vi "Draw.vi"(8 "error in (no error)":errorcluster, 11 "Link in":refnum<class "Link.lvclass">) -> (0 "error out":errorcluster, 2 "Picture":picture, 3 "Link out":refnum<class "Link.lvclass">)   [LabVIEW 2017, in "LV Image Editor Framework.lvlib" / "Link.lvclass"]
uses:
  Link.lvclass
  Line/Line.lvclass
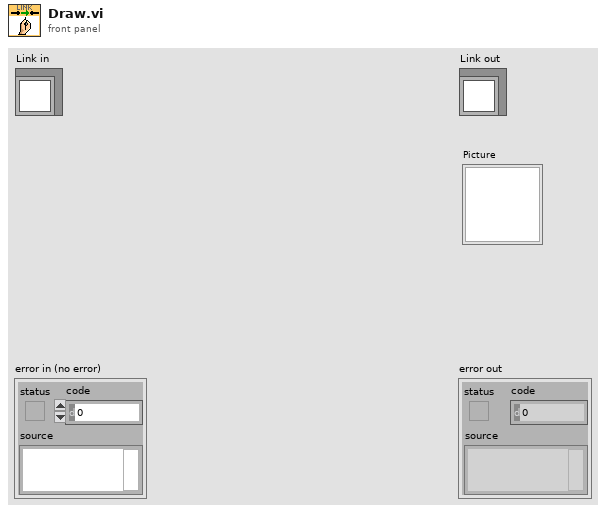
[diagram p1: front panel]
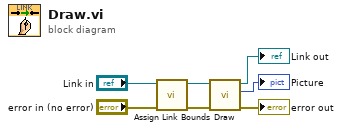
[diagram p0: block diagram]
diagram:
  n1 = call "Assign Link Bounds.vi"("error in (no error)"="error in (no error)", "Link in"="Link in") -> ("error out"=w3:errorcluster, "Link out"=w4:refnum<class "Link.lvclass">)  [unwired: 8 in]
  n2 = call-parent "Draw.vi"("error in (no error)"=w3, "Line in"=w4) -> ("error out"=→"error out":errorcluster, "Picture"=→"Picture":picture, "Line out"=→"Link out":refnum<class "Link.lvclass">)  [unwired: 7 in]
